vi "channel_handle_extended_data.vi"() -> ()   [LabVIEW 2013]
doc: "Illustrates different modes when handling extended data from a SSH server."
uses:
  libssh2/libssh2_init_default.vi
  libssh2/libssh2_session_handshake_tcp.vi
  libssh2/libssh2.lvlib
panel:
  in  "mode (normal)":i32(ring) items=["normal", "ignore", "merge"]
  out "standard error":string
  out "standard output":string
  in  "command":string="echo \"ping: \" && ping localhost -c one"
  in  "password":string
  in  "username":string
  out "error out":errorcluster
  in  "hostname":string="localhost"
  # "This command is deliberately wrong to cause an error!"
  # "Observe the following behavior\n\nmode = normal:\n  The error is reported in \"standard error\"\nmode = ignore:\n  No error is reported (silenced)\nmode = merge:\n  The error is reported in \"standard output\"\n  (together with standard output)"
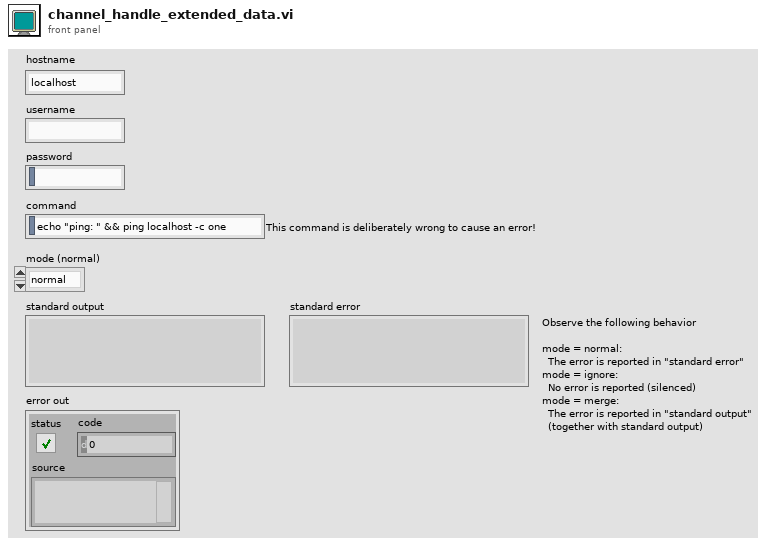
[diagram p1: front panel]
types:
  T1 = typedef "libssh2.lvlib/Session Refnum.ctl" = refnum<k1>
  T2 = typedef "libssh2.lvlib/Channel Refnum.ctl" = refnum<k1>
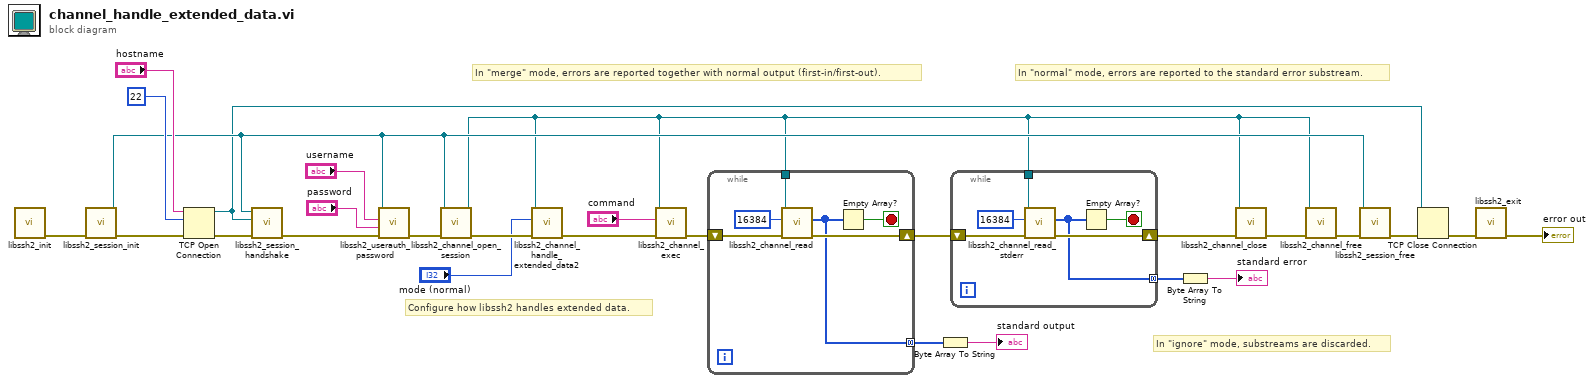
[diagram p0: block diagram]
diagram:
  # "In \"ignore\" mode, substreams are discarded."
  # "In \"merge\" mode, errors are reported together with normal output (first-in/first-out)."
  # "In \"normal\" mode, errors are reported to the standard error substream."
  # "Configure how libssh2 handles extended data."
  n1 = call-poly "libssh2_init.vi"() -> ("error out"=w28:errorcluster)  [unwired: 11 in]
  n2 = call "libssh2_session_init.vi"("error in (no error)"=w28) -> ("error out"=w27:errorcluster, "session"=w13:T1)  [unwired: 9 in]
  n3 = TCP Open Connection(address="hostname", remote port or service name=u16 22, error in (no error)=w27) -> (connection ID=w10:refnum<k5>, error out=w11:errorcluster)  [unwired: 2 in]
  n4 = call-poly "libssh2_session_handshake.vi"("error in (no error)"=w11, "tcp connection"=w10, "session"=w13) -> ("error out"=w5:errorcluster)  [unwired: 8 in]
  n5 = call "libssh2_userauth_password.vi"("error in (no error)"=w5, "password"="password", "username"="username", "session"=w13) -> ("error out"=w22:errorcluster)  [unwired: 7 in]
  n6 = call "libssh2_channel_open_session.vi"("error in (no error)"=w22, "session"=w13) -> ("error out"=w19:errorcluster, "channel"=w2:T2)  [unwired: 8 in]
  n7 = call "libssh2_channel_handle_extended_data2.vi"("error in (no error)"=w19, "mode (normal)"="mode (normal)", "channel"=w2) -> ("error out"=w3:errorcluster)  [unwired: 8 in]
  n8 = call "libssh2_channel_exec.vi"("error in (no error)"=w3, "command"="command", "channel"=w2) -> ("error out"=w18:errorcluster)  [unwired: 8 in]
  n9 = while {
    tunnel: w2 -> [w31]
    tunnel: [w29] -> w15 mode=concatenating
    shift-right: [w33] -> w7
    shift-left: w18 -> [w34]
    stop <- w30 stop-if-true
    n10 = call "libssh2_channel_read.vi"("error in (no error)"=w34, "buffer length"=16384 ("buflen"), "channel"=w31) -> ("error out"=w33:errorcluster, "buffer"=w29:u8[])  [unwired: 7 in]
    n11 = Empty Array?(array=w29) -> (empty?=w30:bool)
  }
  n12 = Byte Array To String(unsigned byte array=w15) -> (string=→"standard output":string)
  n13 = while {
    tunnel: w2 -> [w37]
    tunnel: [w35] -> w8 mode=concatenating
    shift-right: [w39] -> w6
    shift-left: w7 -> [w40]
    stop <- w36 stop-if-true
    n14 = call "libssh2_channel_read_stderr.vi"("error in (no error)"=w40, "buffer length"=16384 ("buflen"), "channel"=w37) -> ("error out"=w39:errorcluster, "buffer"=w35:u8[])  [unwired: 7 in]
    n15 = Empty Array?(array=w35) -> (empty?=w36:bool)
  }
  n16 = Byte Array To String(unsigned byte array=w8) -> (string=→"standard error":string)
  n17 = call "libssh2_channel_close.vi"("error in (no error)"=w6, "channel"=w2) -> ("error out"=w4:errorcluster)  [unwired: 9 in]
  n18 = call "libssh2_channel_free.vi"("error in (no error)"=w4, "channel"=w2) -> ("error out"=w16:errorcluster)  [unwired: 9 in]
  n19 = call "libssh2_session_free.vi"("error in (no error)"=w16, "session"=w13) -> ("error out"=w26:errorcluster)  [unwired: 9 in]
  n20 = TCP Close Connection(connection ID=w10, error in (no error)=w26) -> (error out=w12:errorcluster)  [unwired: 1 in, 1 out]
  n21 = call "libssh2_exit.vi"("error in (no error)"=w12) -> ("error out"=→"error out":errorcluster)  [unwired: 10 in]
